vi "FunctionGenerator.vi"() -> ()   [LabVIEW 2020]
uses:
  rappg_week8/Control 2.ctl
  <vilib>/DAQmx/write.llb/DAQmx Write (Analog 1D DBL 1Chan NSamp).vi
  <vilib>/DAQmx/create/channels.llb/DAQmx Create Channel (AO-Voltage-Basic).vi
  <vilib>/DAQmx/configure/timing.llb/DAQmx Timing (Sample Clock).vi
  <vilib>/DAQmx/miscellaneous.llb/DAQmx Fill In Error Info.vi
  <resource>/objmgr/daqmx.rc
panel:
  out "Actual Freq":dbl
  out "Array Size":dbl
  out "Update Rate":dbl
  in  "physical channels":tag
  in  "stop":bool
  out "Waveform Graph":dbl[](graph)
  in  "Cluster":T1={"Amplitude (V)"=0.0, "Duty Cycle"=0.01, "DC Offset"=0.0, "Waveform"=enum."TTL Wave", "Frequency"=1000.0} {"Frequency" min=1.0 max=100000.0 step=5000.0 format="%#_6p"; "DC Offset" min=-10.0 max=10.0 scale=-10.0..10.0; "Duty Cycle" min=0.01 max=0.99 scale=0.0..1.0; "Amplitude (V)" min=0.0 max=10.0 scale=0.0..10.0}
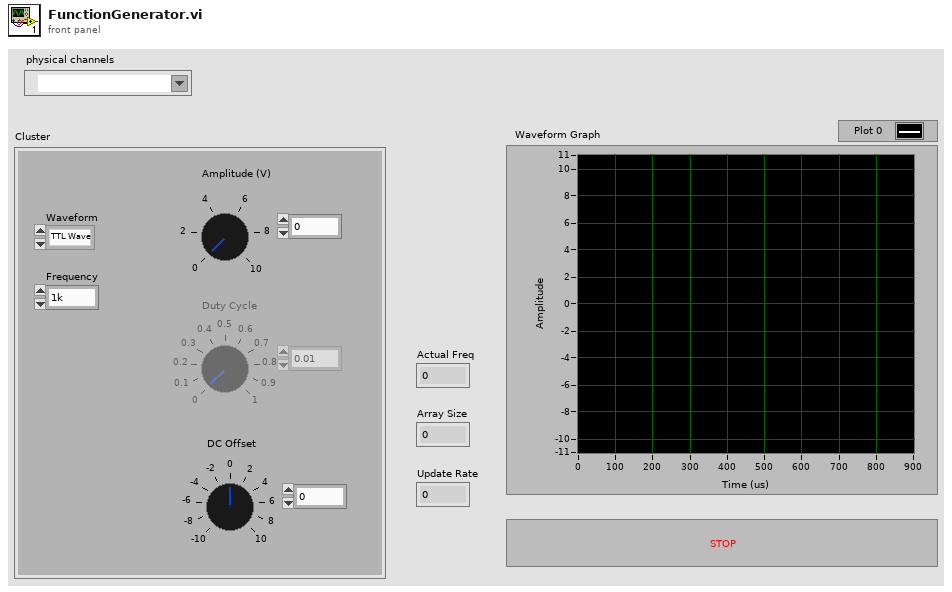
[diagram p1: front panel]
types:
  T1 = cluster{"Amplitude (V)":dbl, "Duty Cycle":dbl, "DC Offset":dbl, "Waveform":enum16{"TTL Wave", "Square Wave", "Sawtooth Wave", "Triangle Wave", "Sine Wave"}, "Frequency":dbl}
  T2 = typedef "Control 2.ctl" = enum16{"Init", "Sine Setup", "TTL Setup", "Sawtooth Setup", "Square Setup", "Triangle Setup", "Wait for GUI", "Stop"}
  T3 = enum16{"TTL Wave", "Square Wave", "Sawtooth Wave", "Triangle Wave", "Sine Wave"}
  T4 = enum8{"Enabled", "Disabled", "Disabled and Grayed Out"}
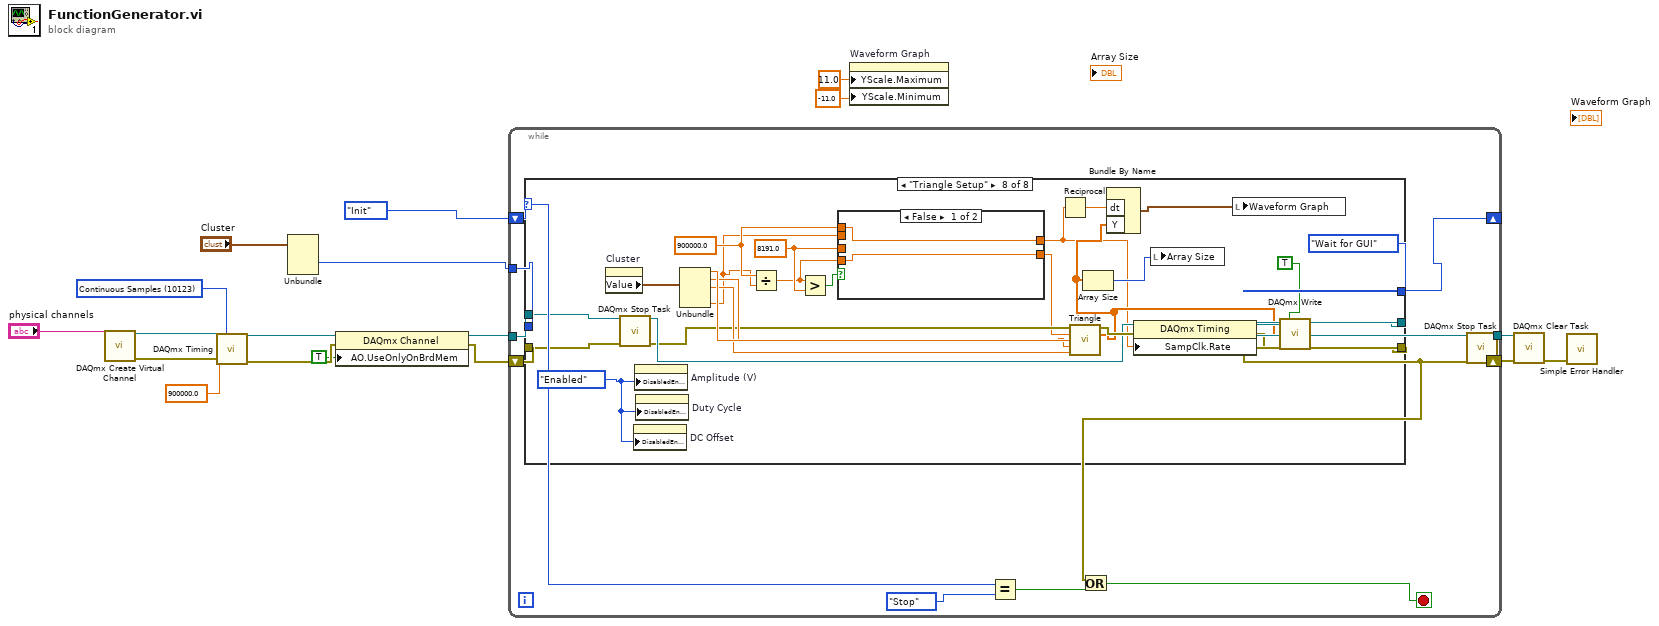
[diagram p0: block diagram]
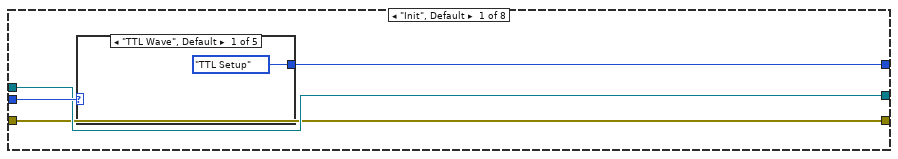
[diagram p2: hidden frame]
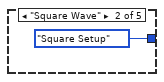
[diagram p3: hidden frame]
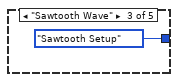
[diagram p4: hidden frame]
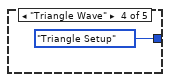
[diagram p5: hidden frame]
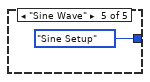
[diagram p6: hidden frame]
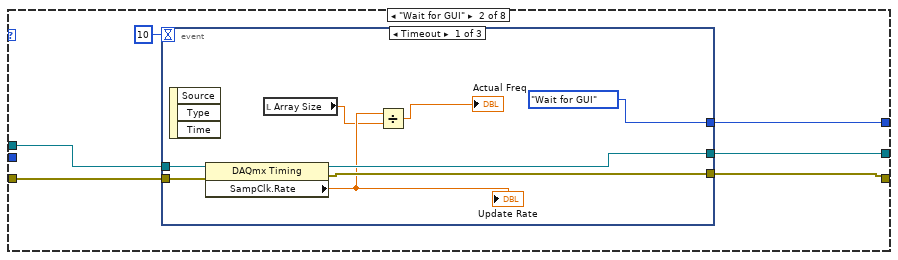
[diagram p7: hidden frame]
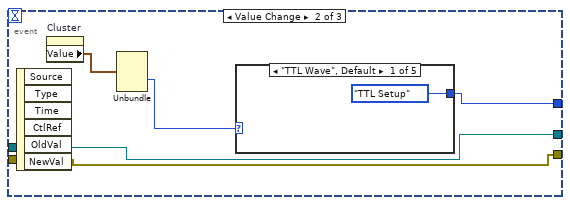
[diagram p8: hidden frame]
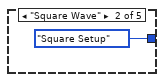
[diagram p9: hidden frame]
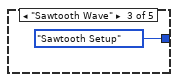
[diagram p10: hidden frame]
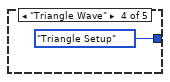
[diagram p11: hidden frame]
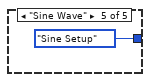
[diagram p12: hidden frame]
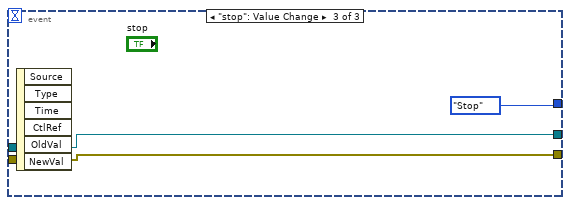
[diagram p13: hidden frame]
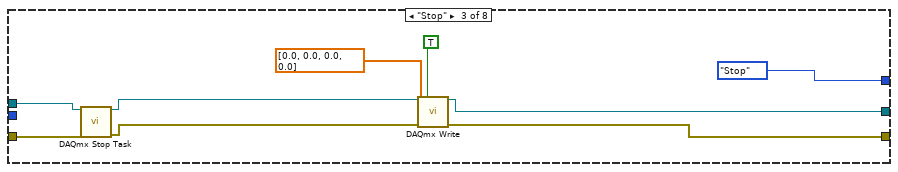
[diagram p14: hidden frame]
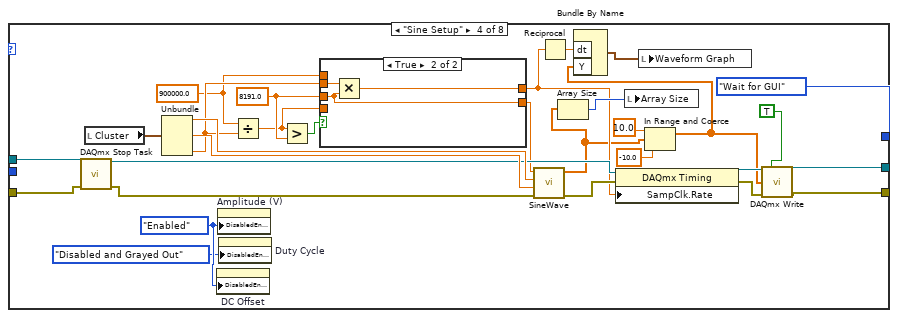
[diagram p15: hidden frame]
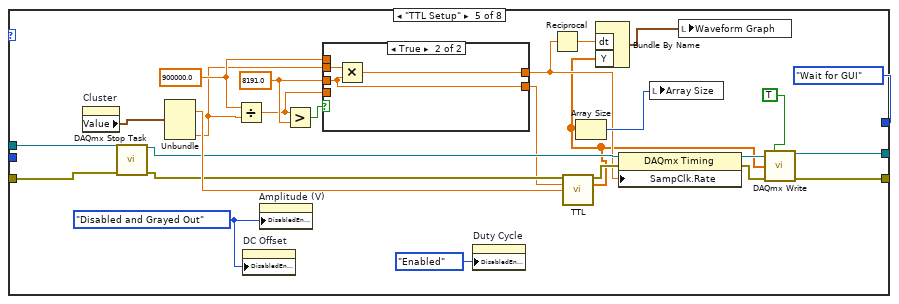
[diagram p17: hidden frame]
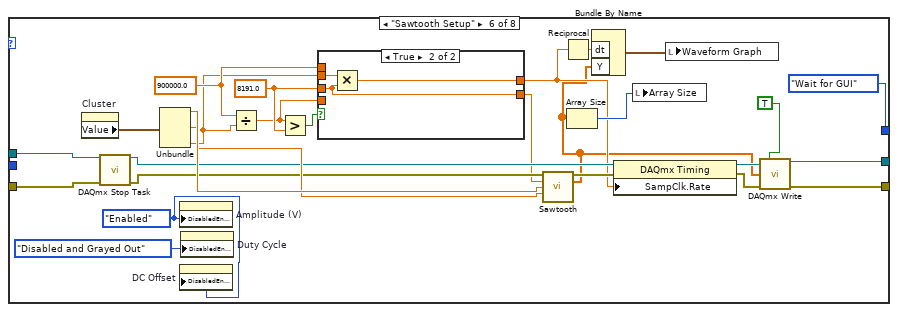
[diagram p19: hidden frame]
diagram:
  w17 = 10123 items=["Finite Samples"=10178, "Continuous Samples"=10123, "Hardware Timed Single Point"=12522] ("sample mode")
  n1 = call-poly <vilib>:"DAQmx Create Virtual Channel.vi"("physical channels"="physical channels") -> ("task out"=w19:refnum<k21>, "error out"=w18:errorcluster)  [unwired: 13 in]
  n2 = call-poly <vilib>:"DAQmx Timing.vi"("task/channels in"=w19, "sample mode"=w17, "rate"=900000.0, "error in"=w18) -> ("task out"=w5:refnum<k21>, "error out"=w4:errorcluster)  [unwired: 10 in]
  n3 = Unbundle("Cluster") -> ("Waveform"=w14:T3)  [unwired: 4 out]
  n4 = property class="DAQmx Channel"(reference=w5, error in=w4, "AO.UseOnlyOnBrdMem"=TRUE) -> (reference out=w7:refnum<k21>, error out=w6:errorcluster)
  n5 = while {
    tunnel: w7 -> [w30]
    tunnel: [w28] -> w12
    shift-right: [w22] -> w11
    shift-left: w6 -> [w29]
    shift-right: [w27] -> _
    shift-left: Control_2."Init" -> [w25]
    tunnel: w14 -> [w26]
    stop <- w21 stop-if-true
    n6 = case shown="\"Triangle Setup\"" w25 {
      tunnel: w26 -> [w34 _ _ _ _ _ _ _]
      tunnel: [w33 w45 Control_2."Stop" Control_2."Wait for GUI" Control_2."Wait for GUI" Control_2."Wait for GUI" Control_2."Wait for GUI" Control_2."Wait for GUI"] -> w27
      tunnel: w30 -> [w32 w44 w69 w93 w123 w154 w185 w216]
      tunnel: w29 -> [w31 w43 w70 w92 w122 w153 w184 w215]
      tunnel: [w31 w41 w72 w104 w125 w155 w187 w222] -> w22
      tunnel: [w32 w42 w73 w103 w126 w156 w188 w223] -> w28
      frame "Init", Default {
        n7 = case shown="\"TTL Wave\", Default" w34 {
          tunnel: [Control_2."TTL Setup" Control_2."Square Setup" Control_2."Sawtooth Setup" Control_2."Triangle Setup" Control_2."Sine Setup"] -> w33
          frame "TTL Wave", Default {
          }
          frame "Square Wave" {
          }
          frame "Sawtooth Wave" {
          }
          frame "Triangle Wave" {
          }
          frame "Sine Wave" {
          }
        }
      }
      frame "Wait for GUI" {
        n8 = event shown="[0] Timeout" {
          selector: _ -> [_ _ _]
          dyn-events: _ -> [_ _ _]
          timeout: 10 -> [_ _ _]
          tunnel: [Control_2."Wait for GUI" w56 Control_2."Stop"] -> w45
          tunnel: w44 -> [w53 w55 w65]
          tunnel: w43 -> [w52 w54 w64]
          tunnel: [w51 w55 w65] -> w42
          tunnel: [w50 w54 w64] -> w41
          event Timeout {
            n9 = event-data() -> ()  [unwired: 1 in, 3 out]
            n10 = property class="DAQmx Timing"(reference=w53, error in=w52) -> (reference out=w51:refnum<k21>, error out=w50:errorcluster, "SampClk.Rate"=w49:dbl)
            "Update Rate" <- w49
            n11 = local read "Array Size"() -> (w48:dbl)
            n12 = Divide(x=w49, y=w48) -> (x/y=→"Actual Freq":dbl)
          }
          event "Cluster.Waveform", "Cluster.Frequency", "Cluster.DC Offset", "Cluster.Duty Cycle", "Cluster.Amplitude (V)": Value Change {
            n13 = event-data() -> ()  [unwired: 1 in, 6 out]
            n14 = property on="Cluster" class="Clust (strict)"() -> ("Value"=w58:T1)  [unwired: 2 in, 2 out]
            n15 = Unbundle(w58) -> ("Waveform"=w57:T3)  [unwired: 4 out]
            n16 = case shown="\"TTL Wave\", Default" w57 {
              tunnel: [Control_2."TTL Setup" Control_2."Square Setup" Control_2."Sawtooth Setup" Control_2."Triangle Setup" Control_2."Sine Setup"] -> w56
              frame "TTL Wave", Default {
              }
              frame "Square Wave" {
              }
              frame "Sawtooth Wave" {
              }
              frame "Triangle Wave" {
              }
              frame "Sine Wave" {
              }
            }
          }
          event "stop": Value Change {
            n17 = event-data() -> ()  [unwired: 1 in, 6 out]
          }
        }
      }
      frame "Stop" {
        n18 = call <vilib>:"DAQmx Stop Task.vi"("task/channels in"=w69, "error in"=w70) -> ("task out"=w68:refnum<k21>, "error out"=w67:errorcluster)  [unwired: 12 in]
        n19 = call-poly <vilib>:"DAQmx Write.vi"("task/channels in"=w68, "auto start"=TRUE, "data"=dbl[] [0.0, 0.0, 0.0, 0.0], "error in"=w67) -> ("task out"=w73:refnum<k21>, "error out"=w72:errorcluster)  [unwired: 9 in, 1 out]
      }
      frame "Sine Setup" {
        w86 = T4."Enabled" ("Disabled")
        w98 = 8191.0 ("y")
        w83 = 900000.0 ("x")
        n20 = call <vilib>:"DAQmx Stop Task.vi"("task/channels in"=w93, "error in"=w92) -> ("task out"=w91:refnum<k21>, "error out"=w90:errorcluster)  [unwired: 12 in]
        n21 = local read "Cluster"() -> (w102:T1)
        n22 = Unbundle(w102) -> ("Amplitude (V)"=w101:dbl, "DC Offset"=w100:dbl, "Frequency"=w97:dbl)  [unwired: 2 out]
        n23 = property on="DC Offset" class="Knob (strict)"("DisabledEnum"=w86) -> ()  [unwired: 2 in, 2 out]
        n24 = property on="Amplitude (V)" class="Knob (strict)"("DisabledEnum"=w86) -> ()  [unwired: 2 in, 2 out]
        n25 = property on="Duty Cycle" class="Knob (strict)"("DisabledEnum"=T4."Disabled and Grayed Out" ("Disabled")) -> ()  [unwired: 2 in, 2 out]
        n26 = Divide(x=w83, y=w97) -> (x/y=w96:dbl)
        n27 = Greater?(x=w96, y=w98) -> (0:w99:bool)
        n28 = case shown="True" w99 {
          tunnel: w98 -> [_ w108]
          tunnel: w97 -> [_ w110]
          tunnel: [w106 w109] -> w82
          tunnel: [w107 w108] -> w89
          tunnel: w96 -> [w107 _]
          tunnel: w83 -> [w106 _]
          frame False {
          }
          frame True {
            n29 = Multiply(x=w110, y=w108) -> (x*y=w109:dbl)
          }
        }
        n30 = call "SineWave.vi"("error in (no error)"=w90, "DC Offset"=w100, "Amplitude"=w101, "Amount of points"=w89) -> ("error out"=w95:errorcluster, "Array"=w77:dbl[])  [unwired: 6 in]
        n31 = Reciprocal(x=w82) -> (1/x=w81:dbl)
        n32 = Array Size(array=w77) -> (size(s)=w84:i32)
        n33 = property class="DAQmx Timing"(reference=w91, error in=w95, "SampClk.Rate"=w82) -> (reference out=w88:refnum<k21>, error out=w87:errorcluster)
        n34 = local write "Array Size"(w84) -> ()
        n35 = In Range and Coerce(upper limit=10.0, x=w77, lower limit=-10.0) -> (coerced(x)=w76:dbl[])  [unwired: 1 out]
        n36 = Bundle By Name("dt"=w81, "Y"=w76) -> (w80:waveform(dbl))  [unwired: 1 in]
        n37 = local write "Waveform Graph"(w80) -> ()
        n38 = call-poly <vilib>:"DAQmx Write.vi"("task/channels in"=w88, "auto start"=TRUE, "data"=w76, "error in"=w87) -> ("task out"=w103:refnum<k21>, "error out"=w104:errorcluster)  [unwired: 9 in, 1 out]
      }
      frame "TTL Setup" {
        w116 = T4."Disabled and Grayed Out" ("Disabled")
        w134 = 8191.0 ("y")
        w132 = 900000.0 ("x")
        n39 = property on="Cluster" class="Clust (strict)"() -> ("Value"=w131:T1)  [unwired: 2 in, 2 out]
        n40 = call <vilib>:"DAQmx Stop Task.vi"("task/channels in"=w123, "error in"=w122) -> ("task out"=w121:refnum<k21>, "error out"=w120:errorcluster)  [unwired: 12 in]
        n41 = Unbundle(w131) -> ("Duty Cycle"=w130:dbl, "Frequency"=w118:dbl)  [unwired: 3 out]
        n42 = Divide(x=w132, y=w118) -> (x/y=w133:dbl)
        n43 = property on="DC Offset" class="Knob (strict)"("DisabledEnum"=w116) -> ()  [unwired: 2 in, 2 out]
        n44 = property on="Amplitude (V)" class="Knob (strict)"("DisabledEnum"=w116) -> ()  [unwired: 2 in, 2 out]
        n45 = Greater?(x=w133, y=w134) -> (0:w135:bool)
        n46 = case shown="True" w135 {
          tunnel: w134 -> [_ w140]
          tunnel: w118 -> [_ w139]
          tunnel: [w137 w141] -> w114
          tunnel: [w138 w140] -> w119
          tunnel: w133 -> [w138 _]
          tunnel: w132 -> [w137 _]
          frame False {
          }
          frame True {
            n47 = Multiply(x=w139, y=w140) -> (x*y=w141:dbl)
          }
        }
        n48 = property on="Duty Cycle" class="Knob (strict)"("DisabledEnum"=T4."Enabled" ("Disabled")) -> ()  [unwired: 2 in, 2 out]
        n49 = Reciprocal(x=w114) -> (1/x=w113:dbl)
        n50 = call "TTL.vi"("error in"=w120, "Amount of Points"=w119, "Duty Cycle"=w130) -> ("error out"=w129:errorcluster, "TTL wave array"=w112:dbl[])  [unwired: 11 in]
        n51 = Array Size(array=w112) -> (size(s)=w115:i32)
        n52 = Bundle By Name("dt"=w113, "Y"=w112) -> (w111:waveform(dbl))  [unwired: 1 in]
        n53 = property class="DAQmx Timing"(reference=w121, error in=w129, "SampClk.Rate"=w114) -> (reference out=w128:refnum<k21>, error out=w127:errorcluster)
        n54 = local write "Array Size"(w115) -> ()
        n55 = local write "Waveform Graph"(w111) -> ()
        n56 = call-poly <vilib>:"DAQmx Write.vi"("task/channels in"=w128, "auto start"=TRUE, "data"=w112, "error in"=w127) -> ("task out"=w126:refnum<k21>, "error out"=w125:errorcluster)  [unwired: 9 in, 1 out]
      }
      frame "Sawtooth Setup" {
        w147 = T4."Enabled" ("Disabled")
        w166 = 8191.0 ("y")
        w164 = 900000.0 ("x")
        n57 = property on="Cluster" class="Clust (strict)"() -> ("Value"=w161:T1)  [unwired: 2 in, 2 out]
        n58 = call <vilib>:"DAQmx Stop Task.vi"("task/channels in"=w154, "error in"=w153) -> ("task out"=w152:refnum<k21>, "error out"=w151:errorcluster)  [unwired: 12 in]
        n59 = Unbundle(w161) -> ("Amplitude (V)"=w159:dbl, "DC Offset"=w158:dbl, "Frequency"=w149:dbl)  [unwired: 2 out]
        n60 = property on="Amplitude (V)" class="Knob (strict)"("DisabledEnum"=w147) -> ()  [unwired: 2 in, 2 out]
        n61 = property on="DC Offset" class="Knob (strict)"("DisabledEnum"=w147) -> ()  [unwired: 2 in, 2 out]
        n62 = property on="Duty Cycle" class="Knob (strict)"("DisabledEnum"=T4."Disabled and Grayed Out" ("Disabled")) -> ()  [unwired: 2 in, 2 out]
        n63 = Divide(x=w164, y=w149) -> (x/y=w165:dbl)
        n64 = Greater?(x=w165, y=w166) -> (0:w167:bool)
        n65 = case shown="True" w167 {
          tunnel: w166 -> [_ w172]
          tunnel: w149 -> [_ w171]
          tunnel: [w169 w173] -> w145
          tunnel: [w170 w172] -> w150
          tunnel: w165 -> [w170 _]
          tunnel: w164 -> [w169 _]
          frame False {
          }
          frame True {
            n66 = Multiply(x=w171, y=w172) -> (x*y=w173:dbl)
          }
        }
        n67 = call "Sawtooth.vi"("error in"=w151, "Amount of Points"=w150, "Amplitude"=w159, "DC Offset"=w158) -> ("error out"=w160:errorcluster, "Array"=w143:dbl[])  [unwired: 10 in]
        n68 = Reciprocal(x=w145) -> (1/x=w144:dbl)
        n69 = Array Size(array=w143) -> (size(s)=w146:i32)
        n70 = Bundle By Name("dt"=w144, "Y"=w143) -> (w142:waveform(dbl))  [unwired: 1 in]
        n71 = property class="DAQmx Timing"(reference=w152, error in=w160, "SampClk.Rate"=w145) -> (reference out=w163:refnum<k21>, error out=w162:errorcluster)
        n72 = local write "Array Size"(w146) -> ()
        n73 = local write "Waveform Graph"(w142) -> ()
        n74 = call-poly <vilib>:"DAQmx Write.vi"("task/channels in"=w163, "auto start"=TRUE, "data"=w143, "error in"=w162) -> ("task out"=w156:refnum<k21>, "error out"=w155:errorcluster)  [unwired: 9 in, 1 out]
      }
      frame "Square Setup" {
        w180 = T4."Enabled" ("Disabled")
        w197 = 8191.0 ("y")
        w195 = 900000.0 ("x")
        n75 = property on="Cluster" class="Clust (strict)"() -> ("Value"=w192:T1)  [unwired: 2 in, 2 out]
        n76 = call <vilib>:"DAQmx Stop Task.vi"("task/channels in"=w185, "error in"=w184) -> ("task out"=w183:refnum<k21>, "error out"=w175:errorcluster)  [unwired: 12 in]
        n77 = property on="Duty Cycle" class="Knob (strict)"("DisabledEnum"=w180) -> ()  [unwired: 2 in, 2 out]
        n78 = property on="Amplitude (V)" class="Knob (strict)"("DisabledEnum"=w180) -> ()  [unwired: 2 in, 2 out]
        n79 = property on="DC Offset" class="Knob (strict)"("DisabledEnum"=w180) -> ()  [unwired: 2 in, 2 out]
        n80 = Unbundle(w192) -> ("Amplitude (V)"=w191:dbl, "Duty Cycle"=w190:dbl, "DC Offset"=w189:dbl, "Frequency"=w181:dbl)  [unwired: 1 out]
        n81 = Divide(x=w195, y=w181) -> (x/y=w196:dbl)
        n82 = Greater?(x=w196, y=w197) -> (0:w198:bool)
        n83 = case shown="True" w198 {
          tunnel: w197 -> [_ w203]
          tunnel: w181 -> [_ w202]
          tunnel: [w200 w204] -> w177
          tunnel: [w201 w203] -> w182
          tunnel: w196 -> [w201 _]
          tunnel: w195 -> [w200 _]
          frame False {
          }
          frame True {
            n84 = Multiply(x=w202, y=w203) -> (x*y=w204:dbl)
          }
        }
        n85 = call "Square.vi"("error in"=w175, "Amount of Points"=w182, "Amplitude"=w191, "Duty Cycle"=w190, "DC Offset"=w189) -> ("error IO"=w174:errorcluster, "Square Wave Array"=w178:dbl[])  [unwired: 9 in]
        n86 = Reciprocal(x=w177) -> (1/x=w176:dbl)
        n87 = Array Size(array=w178) -> (size(s)=w179:i32)
        n88 = Bundle By Name("dt"=w176, "Y"=w178) -> ()  [unwired: 1 in, 1 out]
        n89 = property class="DAQmx Timing"(reference=w183, error in=w174, "SampClk.Rate"=w177) -> (reference out=w194:refnum<k21>, error out=w193:errorcluster)
        n90 = local write "Array Size"(w179) -> ()
        n91 = local write "Waveform Graph"(w178) -> ()
        n92 = call-poly <vilib>:"DAQmx Write.vi"("task/channels in"=w194, "auto start"=TRUE, "data"=w178, "error in"=w193) -> ("task out"=w188:refnum<k21>, "error out"=w187:errorcluster)  [unwired: 9 in, 1 out]
      }
      frame "Triangle Setup" {
        w210 = T4."Enabled" ("Disabled")
        w229 = 8191.0 ("y")
        w227 = 900000.0 ("x")
        n93 = property on="Cluster" class="Clust (strict)"() -> ("Value"=w220:T1)  [unwired: 2 in, 2 out]
        n94 = call <vilib>:"DAQmx Stop Task.vi"("task/channels in"=w216, "error in"=w215) -> ("task out"=w214:refnum<k21>, "error out"=w213:errorcluster)  [unwired: 12 in]
        n95 = property on="DC Offset" class="Knob (strict)"("DisabledEnum"=w210) -> ()  [unwired: 2 in, 2 out]
        n96 = property on="Amplitude (V)" class="Knob (strict)"("DisabledEnum"=w210) -> ()  [unwired: 2 in, 2 out]
        n97 = property on="Duty Cycle" class="Knob (strict)"("DisabledEnum"=w210) -> ()  [unwired: 2 in, 2 out]
        n98 = Unbundle(w220) -> ("Amplitude (V)"=w219:dbl, "Duty Cycle"=w218:dbl, "DC Offset"=w217:dbl, "Frequency"=w211:dbl)  [unwired: 1 out]
        n99 = Divide(x=w227, y=w211) -> (x/y=w228:dbl)
        n100 = Greater?(x=w228, y=w229) -> (0:w230:bool)
        n101 = case shown="False" w230 {
          tunnel: w229 -> [_ w235]
          tunnel: w211 -> [_ w234]
          tunnel: [w232 w236] -> w207
          tunnel: [w233 w235] -> w212
          tunnel: w228 -> [w233 _]
          tunnel: w227 -> [w232 _]
          frame False {
          }
          frame True {
            n102 = Multiply(x=w234, y=w235) -> (x*y=w236:dbl)
          }
        }
        n103 = Reciprocal(x=w207) -> (1/x=w206:dbl)
        n104 = call "Triangle.vi"("error in"=w213, "Amount of Points"=w212, "Amplitude"=w219, "Duty Cycle"=w218, "DC Offset"=w217) -> ("error out"=w221:errorcluster, "Triangle wave array"=w208:dbl[])  [unwired: 9 in]
        n105 = Array Size(array=w208) -> (size(s)=w209:i32)
        n106 = Bundle By Name("dt"=w206, "Y"=w208) -> (w205:waveform(dbl))  [unwired: 1 in]
        n107 = property class="DAQmx Timing"(reference=w214, error in=w221, "SampClk.Rate"=w207) -> (reference out=w226:refnum<k21>, error out=w225:errorcluster)
        n108 = local write "Array Size"(w209) -> ()
        n109 = local write "Waveform Graph"(w205) -> ()
        n110 = call-poly <vilib>:"DAQmx Write.vi"("task/channels in"=w226, "auto start"=TRUE, "data"=w208, "error in"=w225) -> ("task out"=w223:refnum<k21>, "error out"=w222:errorcluster)  [unwired: 9 in, 1 out]
      }
    }
    n111 = Equal?(x=w25, y=Control_2."Stop") -> (x = y?=w23:bool)
    n112 = Or(x=w22, y=w23) -> (x .or. y?=w21:bool)
  }
  n113 = property on="Waveform Graph" class="WFGraph (strict)"("YScale.Maximum"=11.0 ("Y Scale.Range:Maximum"), "YScale.Minimum"=-11.0 ("Y Scale.Range:Minimum")) -> ()  [unwired: 2 in, 2 out]
  n114 = call <vilib>:"DAQmx Stop Task.vi"("task/channels in"=w12, "error in"=w11) -> ("task out"=w10:refnum<k21>, "error out"=w9:errorcluster)  [unwired: 12 in]
  n115 = call <vilib>:"DAQmx Clear Task.vi"("task in"=w10, "error in"=w9) -> ("error out"=w8:errorcluster)  [unwired: 13 in]
  n116 = call <vilib>:"Simple Error Handler.vi"("error in (no error)"=w8) -> ()  [unwired: 4 in, 5 out]
